vi "Get Attribute Name and Parent ID.vi"(8 "error in (no error)":errorcluster, 10 "Tag":string, 11 "Linked List Ref":refnum<data-value>) -> (0 "error out":errorcluster, 1 "Attribute Name":string, 2 "Linked List ID":string, 3 "Linked List Ref out":refnum<data-value>)   [LabVIEW 2020, in "Linked Lists.lvlib" / "Linked List Ref.lvclass"]
uses:
  <vilib>/gpm_packages/@cs/linked-list/Source/Linked List/Linked List Ref/Linked List Ref.lvclass
  <vilib>/gpm_packages/@cs/linked-list/Source/Linked List/ILinkedList/ILinked List.lvclass
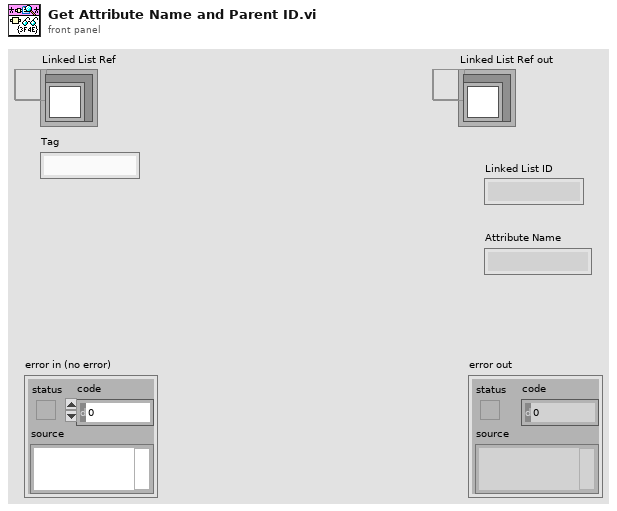
[diagram p1: front panel]
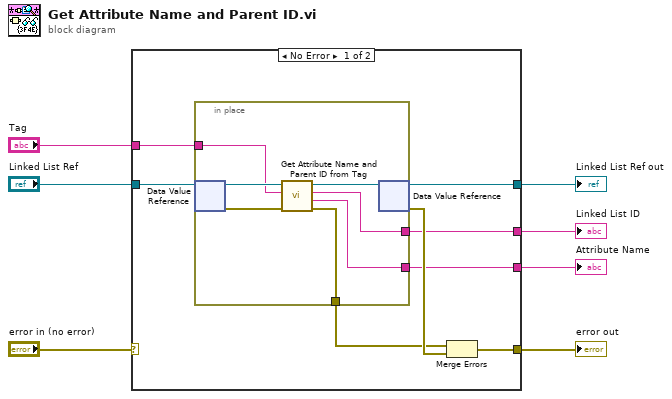
[diagram p0: block diagram]
diagram:
  n1 = case shown="No Error" "error in (no error)" {
    selector: "error in (no error)" -> [_ w24]
    tunnel: "Linked List Ref" -> [w15 w23]
    tunnel: "Tag" -> [w14 _]
    tunnel: [w12 w24] -> w4
    tunnel: [w13 w23] -> w3
    tunnel: [w9 _] -> w2
    tunnel: [w8 _] -> w1
    frame No Error {
      n2 = in-place {
        in-place-border: w14 -> [w20]
        in-place-border: [w18] -> w10
        in-place-border: [w17] -> w9
        in-place-border: [w16] -> w8
        n3 = in-place-dvr #1(w15) -> (w22:refnum<class "ILinked List.lvclass">, w19:errorcluster)
        n4 = call-dynamic "Get Attribute Name and Parent ID from Tag.vi"("error in (no error)"=w19, "Tag"=w20, "ILinked List in"=w22) -> ("error out"=w18:errorcluster, "Attribute Name"=w16:string, "Linked List ID"=w17:string, "ILinked List out"=w21:refnum<class "ILinked List.lvclass">)  [unwired: 5 in]
        n5 = in-place-dvr #1(w21) -> (w13:refnum<data-value>, w11:errorcluster)
      }
      n6 = Merge Errors(w10, w11) -> (w12:errorcluster)
    }
    frame Error {
    }
  }
  "error out" <- w4
  "Linked List Ref out" <- w3
  "Linked List ID" <- w2
  "Attribute Name" <- w1
